vi "Open Session.vi"(0 "instruction target":refnum<class "niInstr Instruction Target v1 Host.lvclass">, 5 "parent context":refnum<class "niInstr Instruction Framework Context v1 Host.lvclass">, 7 "instance(s)":u8[](array[numeric]), 11 "error in":errorcluster, 12 "select session":refnum<class "niHighSpeedSerial Eye Scan Single Point v1 Host.lvclass">) -> (4 "eye scan out":refnum<class "niHighSpeedSerial Rectangular Eye Scan v1 Host.lvclass">, 15 "error out":errorcluster)   [LabVIEW 2016, in "niHighSpeedSerial Rectangular Eye Scan v1 Host.lvclass"]
doc: "Opens a session to Eye Scan and reserves resources.\n\n<B>Input Parameters</B>\n\n<B>instruction target</B> is the instruction target to use when communicating with the FPGA.\n\n<B>parent context</B> is the context of the parent instance. In most cases you can wire a default value.\n\n<B>instance(s)</B> The channel instances used.\n\n<B>error in</B> describes error conditions that occur before this node runs. This input provides standard 'error in' functionality.\n\n<B>Output Parameters</B>\n\n<B>eye scan out</B> passes a reference to your session to the next VI.\n\n<B>error out</B> contains error information. This output provides standard 'error out' functionality."
uses:
  <instrlib>/niHighSpeedSerial/Eye Scan/v1/Host/Impl/Rectangular Eye Scan/niHighSpeedSerial Rectangular Eye Scan v1 Host.lvclass
  C:/Penguin/dasplund-dasplund/lvdist/win32/export/16.0/16.0.0f0/dist/instr.lib/niHighSpeedSerial/Eye Scan/v1/Host/Eye Scan/niHighSpeedSerial Eye Scan v1 Host.lvclass
  <instrlib>/_niInstr/Instruction Framework/v1/Host/Instruction Framework Context/niInstr Instruction Framework Context v1 Host.lvclass
  <instrlib>/_niInstr/Instruction Framework/v1/Host/Instruction Target/niInstr Instruction Target v1 Host.lvclass
  <instrlib>/niHighSpeedSerial/Eye Scan/v1/Host/Impl/Single Point/niHighSpeedSerial Eye Scan Single Point v1 Host.lvclass
  <instrlib>/niHighSpeedSerial/Eye Scan/v1/Host/Impl/Rectangular Eye Scan/Private/Private Data.ctl
  <instrlib>/niHighSpeedSerial/Eye Scan/v1/Host/Impl/Rect Iter/niHighSpeedSerial Rectangular Eye Scan Point Iterator v1 Host.lvclass
  <instrlib>/niHighSpeedSerial/Eye Scan/v1/Host/Impl/Rectangular Eye Scan/niHighSpeedSerial Rectangular Eye Scan v1 Host.lvclass/niHighSpeedSerial Rectangular Eye Scan v1 Host.ctl
  <instrlib>/niHighSpeedSerial/Eye Scan/v1/Host/Eye Scan/niHighSpeedSerial Eye Scan v1 Host.lvclass
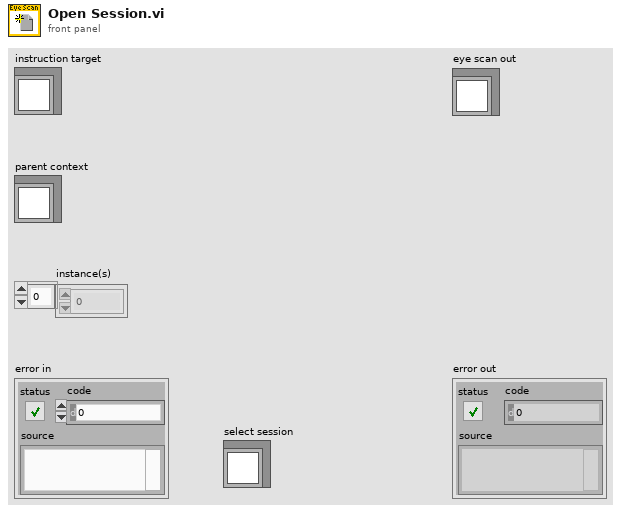
[diagram p1: front panel]
types:
  T1 = typedef "niHighSpeedSerial Rectangular Eye Scan v1 Host.lvclass/Private Data.ctl" = cluster{"horizontal step size":i16, "vertical step size":i16, "rectangular eye scan point iterator":refnum<class "niHighSpeedSerial Rectangular Eye Scan Point Iterator v1 Host.lvclass">}
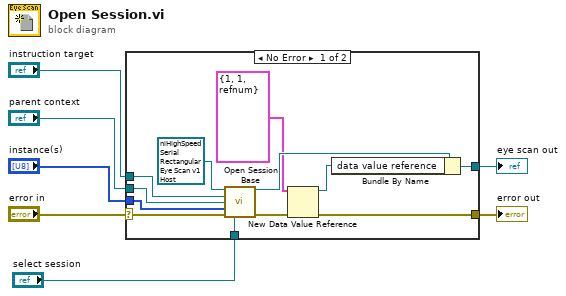
[diagram p0: block diagram]
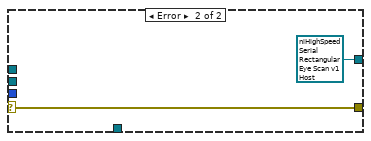
[diagram p2: hidden frame]
diagram:
  n1 = case shown="No Error" "error in" {
    selector: "error in" -> [w16 w21]
    tunnel: [w10 w21] -> w6
    tunnel: "parent context" -> [w17 _]
    tunnel: "instruction target" -> [w19 _]
    tunnel: "instance(s)" -> [w15 _]
    tunnel: [w13 refnum<class "niHighSpeedSerial Rectangular Eye Scan v1 Host.lvclass"> refnum ("Rectangular Eye Scan v1 Host out")] -> w2
    tunnel: "select session" -> [w8 _]
    frame No Error {
      n2 = call <instrlib>:"Open Session Base.vi"("eye scan in"=refnum<class "niHighSpeedSerial Rectangular Eye Scan v1 Host.lvclass"> refnum ("Rectangular Eye Scan v1 Host out"), "instruction target"=w19, "parent context"=w17, "instance(s)"=w15, "error in"=w16, "select session"=w8) -> ("eye scan out"=w14:refnum<class "niHighSpeedSerial Rectangular Eye Scan v1 Host.lvclass">, "error out"=w12:errorcluster)  [unwired: 8 in]
      n3 = New Data Value Reference(data value=T1 {"horizontal step size"=1, "vertical step size"=1, "rectangular eye scan point iterator"=refnum} ("private data"), error in=w12) -> (data value reference=w11:refnum<data-value>, error out=w10:errorcluster)
      n4 = Bundle By Name(cluster=w14, "data value reference"=w11) -> (w13:refnum<class "niHighSpeedSerial Rectangular Eye Scan v1 Host.lvclass">)
    }
    frame Error {
    }
  }
  "error out" <- w6
  "eye scan out" <- w2
